vi "LED2.vi"() -> ()   [LabVIEW 2024]
uses:
  <vilib>/LabVIEW Interface for Arduino/LabVIEW Interface for Arduino.lvlib
panel:
  in  "Digital I/O Pin (0)":u8
  in  "VISA resource":refnum<visa-resource-name>
  in  "stop":bool
  in  "เปิด/ปิด":bool
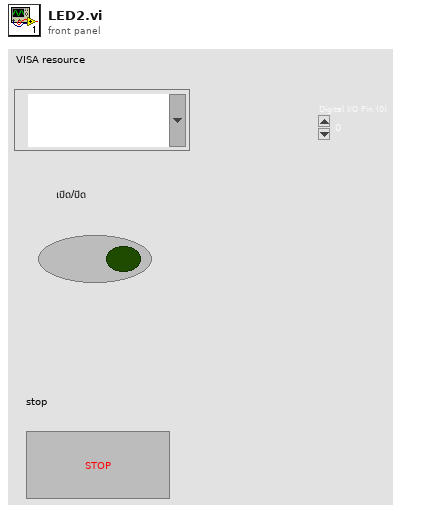
[diagram p1: front panel]
types:
  T1 = typedef "LabVIEW Interface for Arduino.lvlib/Arduino Resource.ctl" = cluster{"VISA resource":refnum<visa-resource-name>, "Board Type":T2, "Connection Type":enum8{"USB / Serial"}, "Bytes Per Packet (15)":u8}
  T2 = typedef "LabVIEW Interface for Arduino.lvlib/Board Type.ctl" = enum16{"Uno", "Dimuelanove w/Atmega 328", "Mega 2560"}
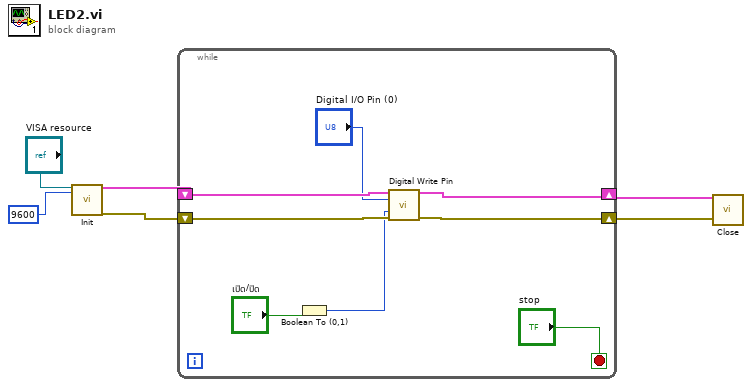
[diagram p0: block diagram]
diagram:
  n1 = call <vilib>:"Init.vi"("VISA resource"="VISA resource", "Baud Rate (115200)"=u32 9600) -> ("Arduino Resource"=w6:T1, "error out"=w5:errorcluster)  [unwired: 16 in]
  n2 = while {
    shift-right: [w10] -> w3
    shift-left: w6 -> [w13]
    shift-right: [w11] -> w4
    shift-left: w5 -> [w12]
    stop <- "stop" stop-if-true
    n3 = Boolean To (0,1)(Boolean="เปิด/ปิด") -> (0, 1=w7:i16)
    n4 = call <vilib>:"Digital Write Pin.vi"("Arduino Resource"=w13, "Digital I/O Pin (0)"="Digital I/O Pin (0)", "Value (0)"=w7, "error in"=w12) -> ("Arduino Resource"=w10:T1, "error out"=w11:errorcluster)  [unwired: 10 in]
  }
  n5 = call <vilib>:"Close.vi"("Arduino Resource"=w3, "error in"=w4) -> ()  [unwired: 13 in, 1 out]
